vi "Configure Serial Port.vi"(5 "Timeout":u32=10000, 6 "flow control":u16(ring) items=["None", "XON/XOFF", "RTS/CTS", "XON/XOFF & RTS/CTS", "DTR/DSR", "XON/XOFF & DTR/DSR"], 7 "data bits":u16, 8 "error in (no error)":errorcluster, 9 "parity":u16(ring)=2 items=["None", "Odd", "Even", "Mark", "Space"], 10 "baud rate":u32=9600, 11 "VISA refnum in":refnum<visa-resource-name>) -> (0 "error out":errorcluster)   [LabVIEW 2018, in "SubVIs.lvlib" / "Serial Shared Components.lvlib"]
doc: "Configures a selected serial port with various options."
uses:
  Serial Shared Components.lvlib
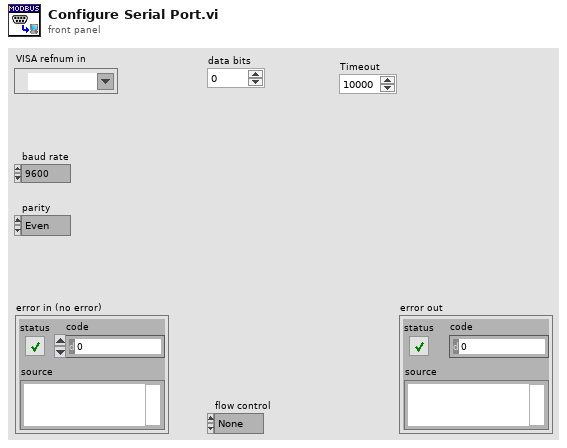
[diagram p1: front panel]
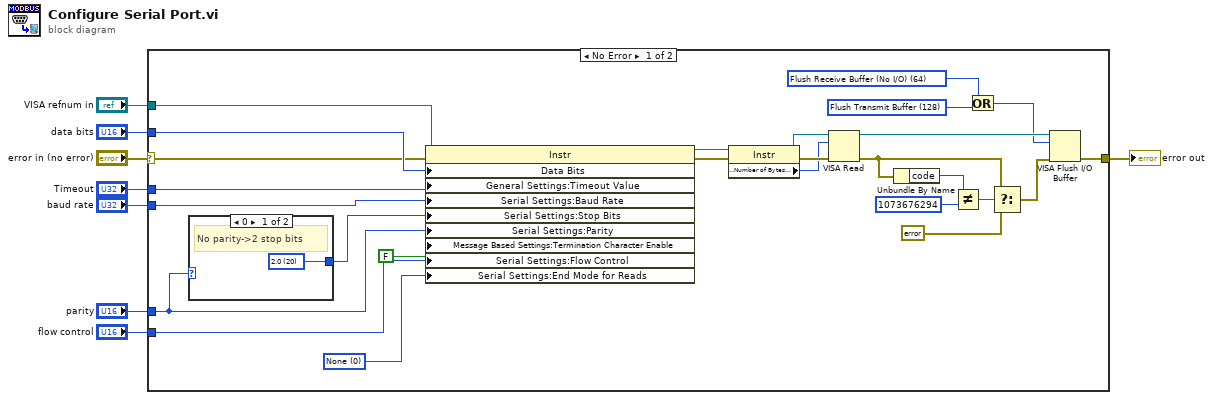
[diagram p0: block diagram]
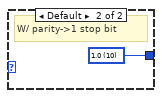
[diagram p2: hidden frame]
diagram:
  n1 = case shown="No Error" "error in (no error)" {
    selector: "error in (no error)" -> [w10 w37]
    tunnel: "data bits" -> [w34 _]
    tunnel: [w33 w37] -> w7
    tunnel: "VISA refnum in" -> [w32 _]
    tunnel: "baud rate" -> [w23 _]
    tunnel: "flow control" -> [w18 _]
    tunnel: "parity" -> [w17 _]
    tunnel: "Timeout" -> [w9 _]
    frame No Error {
      w22 = u16 128 items=["Flush Receive Buffer"=16, "Write Transmit Buffer to Device"=32, "Flush Receive Buffer (No I/O)"=64, "Flush Transmit Buffer"=128] ("Mask")
      w21 = u16 64 items=["Flush Receive Buffer"=16, "Write Transmit Buffer to Device"=32, "Flush Receive Buffer (No I/O)"=64, "Flush Transmit Buffer"=128] ("Mask")
      w24 = u16 0 items=["None", "LastBit", "TermChar"] ("Serial Settings:Serial End Mode for Reads")
      n2 = case "http://modbus.org/docs/Modbus_over_serial_line_V1_02.pdf" shown="0" w17 {
        tunnel: [w35 w36] -> w19
        frame 0 {
          w35 = u16 20 items=["1.0"=10, "1.5"=15, "2.0"=20] ("Serial Settings:Serial Stop Bits")
          # "No parity->2 stop bits"
        }
        frame Default {
          w36 = u16 10 items=["1.0"=10, "1.5"=15, "2.0"=20] ("Serial Settings:Serial Stop Bits")
          # "W/ parity->1 stop bit"
        }
      }
      n3 = property class="Instr"(reference=w32, error in=w10, "Data Bits"=w34, "General Settings:Timeout Value"=w9, "Serial Settings:Baud Rate"=w23, "Serial Settings:Stop Bits"=w19, "Serial Settings:Parity"=w17, "Message Based Settings:Termination Character Enable"=FALSE, "Serial Settings:Flow Control"=w18, "Serial Settings:End Mode for Reads"=w24) -> (reference out=w27:refnum<visa-resource-name>, error out=w26:errorcluster)
      n4 = property class="Instr"(reference=w27, error in=w26) -> (reference out=w29:refnum<visa-resource-name>, error out=w31:errorcluster, "Serial Settings:Number of Bytes at Serial Port"=w30:u32)
      n5 = VISA Read(VISA resource name=w29, byte count=w30, error in (no error)=w31) -> (VISA resource name out=w28:refnum<visa-resource-name>, error out=w13:errorcluster)  [unwired: 2 out]
      n6 = Unbundle By Name(w13) -> ("code"=w16:i32)
      n7 = Not Equal?(x=w16, y=1073676294) -> (x != y?=w14:bool)
      n8 = Or(x=w21, y=w22) -> (x .or. y?=w20:u16)
      n9 = Select(t=w13, s=w14, f=errorcluster {"status"=FALSE, "code"=0, "source"=""}) -> (s? t:f=w11:errorcluster)
      n10 = VISA Flush I/O Buffer(VISA resource name=w28, mask (16)=w20, error in (no error)=w11) -> (error out=w33:errorcluster)  [unwired: 1 out]
    }
    frame Error {
    }
  }
  "error out" <- w7
